vi "Get CD Properties.vi"(8 "error in (no error)":errorcluster, 11 "Device Reference in":T1 format="%.0x") -> (0 "error out":errorcluster, 2 "Section Properties":T2={"CAN"={"Database File"=path "", "CAN Interface"=enum."CAN0", "Baud Rate"=0, "Diagnostic Protocol"=enum."GMLAN", "Transport Protocol"=enum."ISO TP - Normal Mode", "Transmit ID"=0, "Receive ID"=0, "Transmit Extension"=0, "Receive Extension"=0, "Receive UUDT ID"=0, "Enable Stream"=TRUE, "VW TP Channel ID"=0, "Security"={"DLL Path"=path "", "Security Level"=1}}, "DPIDs"=[], "DTC descriptor"={"DTC Byte Length"=2, "Status Byte Length"=1, "Add Data Byte Length"=1, "Byte Order"=enum."Motorola"}, "PIDs"=[], "DIDs"=[], "CPIDs"=[]} {"CPIDs"."Signals"."Byte Order" items=["Little Endian", "Big Endian"]; "CPIDs"."Signals"."Data Type" items=["Signed", "Unsigned", "IEEE Float"]; "DIDs"."Signals"."Byte Order" items=["Little Endian", "Big Endian"]; "DIDs"."Signals"."Data Type" items=["Signed", "Unsigned", "IEEE Float"]; "CAN"."VW TP Channel ID" format="%.0x"; "CAN"."Receive UUDT ID" format="%.0x"; "CAN"."Receive Extension" format="%.0x"; "CAN"."Transmit Extension" format="%.0x"; "CAN"."Receive ID" format="%.0x"; "CAN"."Transmit ID" format="%.0x"; "PIDs"."Signals"."Byte Order" items=["Little Endian", "Big Endian"]; "PIDs"."Signals"."Data Type" items=["Signed", "Unsigned", "IEEE Float"]}, 3 "Device Reference out":T1 format="%.0x")   [LabVIEW 2015, in "Diagnostics Addon Engine.lvlib"]
uses:
  Diagnostics Addon Engine.lvlib
  <vilib>/NI Veristand/Custom Device API/Custom Device Item Ref.ctl
  Section Properties.ctl
  Shared/CAN Configuration.ctl
  Shared/CAN Interface.ctl
  Shared/Diagnostic Protocols.ctl
  Shared/Transport Protocols.ctl
  Shared/Security.ctl
  Shared/DPID Parameters.ctl
  Shared/DPID Periodic Rate.ctl
  <vilib>/Automotive Diagnostic Command Set/Diagnostic Protocols.llb/DTC Descriptor.ctl
  Shared/DIDPID Parameters.ctl
  Shared/DIDPID Signal Parameters.ctl
  Shared/FG Action.ctl
  Shared/Get DIDPID.vi
  Shared/DIDPID ID FG.vi
  Shared/Get Signals from DIDPID.vi
  Shared/Signal Parameters FG.vi
  <vilib>/NI Veristand/Custom Device API/NI VeriStand - Get Custom Device Channel Data.vi
  <vilib>/NI Veristand/Custom Device API/NI VeriStand - Get Item Description.vi
  <vilib>/NI Veristand/Custom Device API/NI VeriStand - Get Item Property.vi
  <vilib>/NI Veristand/Custom Device API/Get Item Property (Variant).vi
  <vilib>/NI Veristand/Custom Device API/NI VeriStand - Set Item Property.vi
  <vilib>/NI Veristand/Custom Device API/Set Item Property (Variant).vi
  Shared/GUID Lookup.vi
  <vilib>/NI Veristand/Custom Device API/NI VeriStand - Get Item Data.vi
  <vilib>/NI Veristand/Custom Device Tools/Custom Device Utility Library/NI VeriStand - Search for Item by GUID.vi
  Shared/Diagnostics Addon Shared.lvlib
  <vilib>/NI Veristand/Custom Device Tools/Custom Device Utility Library/Custom Device Utility Library.lvlib
  <vilib>/NI Veristand/Custom Device API/Custom Device API.lvlib
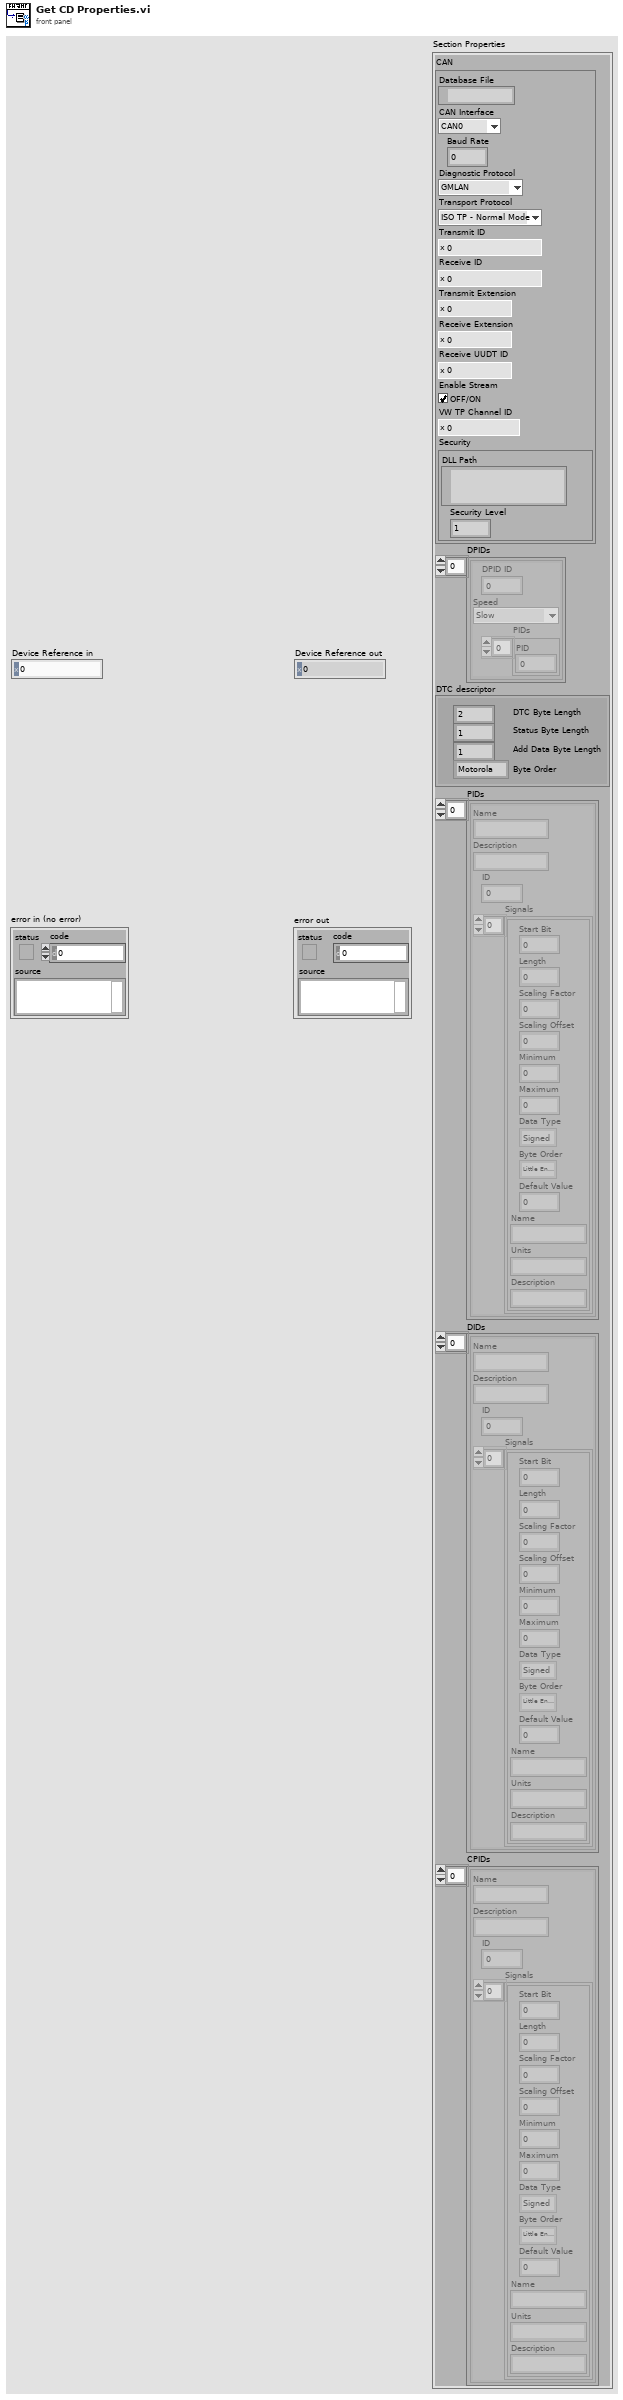
[diagram p1: front panel]
types:
  T1 = typedef "Custom Device API.lvlib/Custom Device Item Ref.ctl" = u64
  T2 = typedef "Diagnostics Addon Engine.lvlib/Section Properties.ctl" = cluster{"CAN":T3, "DPIDs":T8[], "DTC descriptor":T10, "PIDs":T11[], "DIDs":T11[], "CPIDs":T11[]}
  T3 = typedef "Diagnostics Addon Shared.lvlib/CAN Configuration.ctl" = cluster{"Database File":path, "CAN Interface":T4, "Baud Rate":u32, "Diagnostic Protocol":T5, "Transport Protocol":T6, "Transmit ID":u32, "Receive ID":u32, "Transmit Extension":u8, "Receive Extension":u8, "Receive UUDT ID":u32, "Enable Stream":bool, "VW TP Channel ID":u32, "Security":T7}
  T4 = typedef "Diagnostics Addon Shared.lvlib/CAN Interface.ctl" = enum16{"CAN0", "CAN1", "CAN2", "CAN3", "CAN4", "CAN5", "CAN6", "CAN7", "CAN8", "CAN9", "CAN10", "CAN11", "CAN12", "CAN13", "CAN14", "CAN15", "CAN16", "CAN17", "CAN18", "CAN19", "CAN20", "CAN21", "CAN22", "CAN23", "CAN24", "CAN25", "CAN26", "CAN27", "CAN28", "CAN29", "CAN30", "CAN31", "CAN32", "CAN33", "CAN34", "CAN35", "CAN36", "CAN37", "CAN38", "CAN39", "CAN40", "CAN41", "CAN42", "CAN43", "CAN44", "CAN45", "CAN46", "CAN47", "CAN48", "CAN49", "CAN50", "CAN51", "CAN52", "CAN53", "CAN54", "CAN55", "CAN56", "CAN57", "CAN58", "CAN59", "CAN60", "CAN61", "CAN62", "CAN63", "CAN 256 (Virtual)", "CAN 257 (Virtual)"}
  T5 = typedef "Diagnostics Addon Shared.lvlib/Diagnostic Protocols.ctl" = enum16{"GMLAN", "KWP-2000", "UDS"}
  T6 = typedef "Diagnostics Addon Shared.lvlib/Transport Protocols.ctl" = enum16{"ISO TP - Normal Mode", "ISO TP - Mixed Mode", "VW TP 2.0", "Diagnostics on IP"}
  T7 = typedef "Diagnostics Addon Shared.lvlib/Security.ctl" = cluster{"DLL Path":path, "Security Level":u8}
  T8 = typedef "Diagnostics Addon Shared.lvlib/DPID Parameters.ctl" = cluster{"DPID ID":u8, "Speed":T9, "PIDs":u16[]}
  T9 = typedef "Diagnostics Addon Shared.lvlib/DPID Periodic Rate.ctl" = enum16{"Slow", "Medium", "Fast"}
  T10 = typedef "DTC Descriptor.ctl" = cluster{"DTC Byte Length":i32, "Status Byte Length":i32, "Add Data Byte Length":i32, "Byte Order":enum16{"Motorola", "Intel"}}
  T11 = typedef "Diagnostics Addon Shared.lvlib/DIDPID Parameters.ctl" = cluster{"Name":string, "Description":string, "ID":u16, "Signals":T12[]}
  T12 = typedef "Diagnostics Addon Shared.lvlib/DIDPID Signal Parameters.ctl" = cluster{"Start Bit":u8, "Length":u8, "Scaling Factor":dbl, "Scaling Offset":dbl, "Minimum":dbl, "Maximum":dbl, "Data Type":u32, "Byte Order":u32, "Default Value":dbl, "Name":string, "Units":string, "Description":string}
  T13 = typedef "Diagnostics Addon Shared.lvlib/FG Action.ctl" = enum16{"Get", "Set"}
  T14 = enum16{"open", "replace", "create", "open or create", "replace or create", "replace or create with confirmation"}
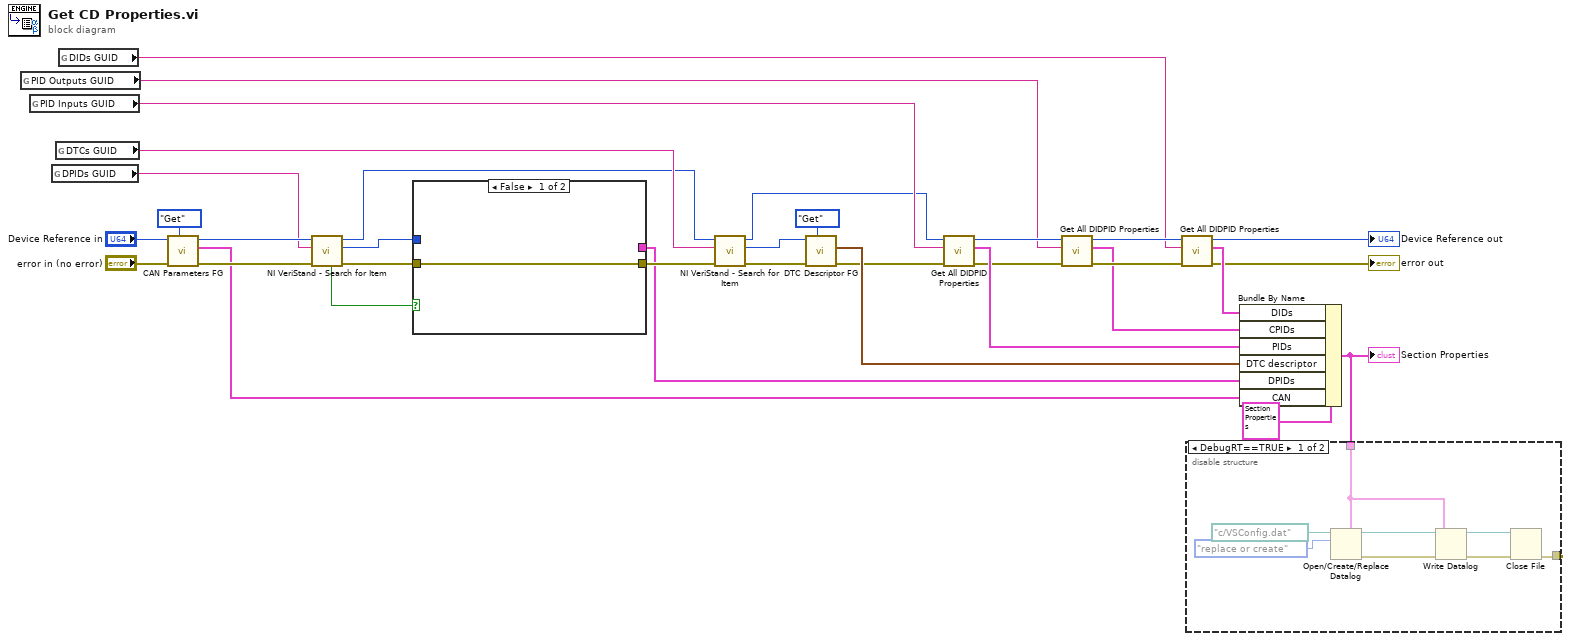
[diagram p0: block diagram]
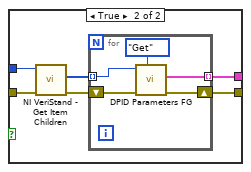
[diagram p2: hidden frame]
diagram:
  n1 = global read "GUID Lookup.vi" "PID Outputs GUID"() -> (w11:string)
  n2 = global read "GUID Lookup.vi" "PID Inputs GUID"() -> (w16:string)
  n3 = global read "GUID Lookup.vi" "DPIDs GUID"() -> (w29:string)
  n4 = global read "GUID Lookup.vi" "DTCs GUID"() -> (w26:string)
  n5 = global read "GUID Lookup.vi" "DIDs GUID"() -> (w8:string)
  n6 = call "CAN Parameters FG.vi"("Action"=FG_Action."Get", "error in (no error)"="error in (no error)", "Device Item Ref in"="Device Reference in") -> ("error out"=w32:errorcluster, "Diagnostics Basic Configuraiton"=w19:T3, "Device Item Ref out"=w31:T1)  [unwired: 6 in]
  n7 = call-poly <vilib>:"NI VeriStand - Search for Item.vi"("error in"=w32, "Item GUID"=w29, "Section Ref in"=w31) -> ("error out"=w30:errorcluster, "Item Ref"=w28:T1, "Section Ref out"=w25:T1, "Found"=w4:bool)  [unwired: 5 in]
  n8 = case shown="False" w4 {
    tunnel: w30 -> [w35 w41]
    tunnel: w28 -> [_ w38]
    tunnel: [w35 w37] -> w27
    tunnel: [_ w36] -> w20
    frame False {
    }
    frame True {
      n9 = call <vilib>:"NI VeriStand - Get Item Children.vi"("error in (no error)"=w41, "Item Ref in"=w38) -> ("error out"=w40:errorcluster, "Child Refs"=w39:T1[])  [unwired: 6 in, 2 out]
      n10 = for {
        tunnel: w39 -> [w45] mode=indexing
        tunnel: [w44] -> w36 mode=indexing
        shift-right: [w43] -> w37
        shift-left: w40 -> [w46]
        n11 = call "DPID Parameters FG.vi"("Action"=FG_Action."Get", "error in (no error)"=w46, "Device Item Ref in"=w45) -> ("error out"=w43:errorcluster, "DPID"=w44:T8)  [unwired: 6 in, 1 out]
      }
    }
  }
  n12 = call-poly <vilib>:"NI VeriStand - Search for Item.vi"("error in"=w27, "Item GUID"=w26, "Section Ref in"=w25) -> ("error out"=w23:errorcluster, "Item Ref"=w24:T1, "Section Ref out"=w3:T1)  [unwired: 5 in, 1 out]
  n13 = call "DTC Descriptor FG.vi"("Action"=FG_Action."Get", "error in (no error)"=w23, "Device Item Ref in"=w24) -> ("error out"=w1:errorcluster, "DTC descriptor"=w21:T10)  [unwired: 6 in, 1 out]
  n14 = call "Get All DIDPID Properties.vi"("error in (no error)"=w1, "PID Inputs GUID"=w16, "Section Ref out in"=w3) -> ("error out"=w15:errorcluster, "DIDPID Array"=w22:T11[], "Section Ref out"=w13:T1)  [unwired: 6 in]
  n15 = call "Get All DIDPID Properties.vi"("error in (no error)"=w15, "PID Inputs GUID"=w11, "Section Ref out in"=w13) -> ("error out"=w14:errorcluster, "DIDPID Array"=w10:T11[], "Section Ref out"=w12:T1)  [unwired: 6 in]
  n16 = call "Get All DIDPID Properties.vi"("error in (no error)"=w14, "PID Inputs GUID"=w8, "Section Ref out in"=w12) -> ("error out"=→"error out":errorcluster, "DIDPID Array"=w9:T11[], "Section Ref out"=→"Device Reference out":T1)  [unwired: 6 in]
  n17 = Bundle By Name(cluster=T2 {"CAN"={"Database File"=path "", "CAN Interface"=enum."CAN0", "Baud Rate"=0, "Diagnostic Protocol"=enum."GMLAN", "Transport Protocol"=enum."ISO TP - Normal Mode", "Transmit ID"=0, "Receive ID"=0, "Transmit Extension"=0, "Receive Extension"=0, "Receive UUDT ID"=0, "Enable Stream"=FALSE, "VW TP Channel ID"=0, "Security"={"DLL Path"=path "", "Security Level"=1}}, "DPIDs"=[], "DTC descriptor"={"DTC Byte Length"=2, "Status Byte Length"=1, "Add Data Byte Length"=1, "Byte Order"=enum."Motorola"}, "PIDs"=[], "DIDs"=[], "CPIDs"=[]} ("input cluster"), "DIDs"=w9, "CPIDs"=w10, "PIDs"=w22, "DTC descriptor"=w21, "DPIDs"=w20, "CAN"=w19) -> (w17:T2)
  "Section Properties" <- w17
  n18 = disable-structure shown="DebugRT==TRUE" {
    disable-tunnel: w17 -> [w50 _]
    disable-tunnel: [w47 _] -> _
    frame condition #0 {
      n19 = Open/Create/Replace Datalog(5:w50, 10:T14."replace or create" ("operation (0:open)"), 11:path "c:/VSConfig.dat" ("datalog path (use dialog)")) -> (0:w52:errorcluster, 3:w53:refnum<k1>)  [unwired: 3 in, 1 out]
      n20 = Write Datalog(4:w52, 6:w50, 7:w53) -> (0:w51:errorcluster, 3:w54:refnum<k1>)
      n21 = Close File(refnum=w54, error in=w51) -> (error out=w47:errorcluster)  [unwired: 1 out]
    }
    frame condition #1 (active) {
    }
  }
